vi "Move Window (hwnd).vi"(8 "error in (no error)":errorcluster, 9 "New Position (0,0)":cluster{"left":i16, "top":i16}, 10 "Window Name (\"\")":string, 11 "HWnd":u32) -> (0 "error out":errorcluster, 1 "Prev Position":cluster{"left":i16, "top":i16}, 3 "HWnd Out":u32)   [LabVIEW 2011]
doc: "This function will move the window named in the 'window name' input or identified by the 'window refnum' from its present location to that defined in the 'new position' cluster. Coordinates are pixels relative to upper left corner of the screen.\n\nIf the function is successful, then:\n'window refnum out' = 'window refnum' if window refnum in is valid;\n'window refnum out' is a new window refnum if 'window refnum' is not valid and 'window name' a valid name for a window.\n\nIf the window cannot be found, an error will be returned and window refnum out will be 'Not a Valid Window RefNum'."
uses:
  user32.dll
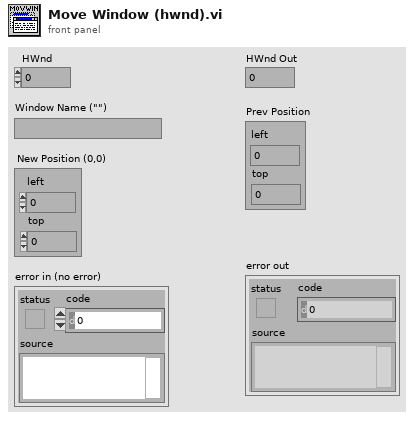
[diagram p1: front panel]
types:
  T1 = typedef "Window Rectangle (hwnd).ctl" = cluster{"left":i16, "top":i16, "right":i16, "bottom":i16}
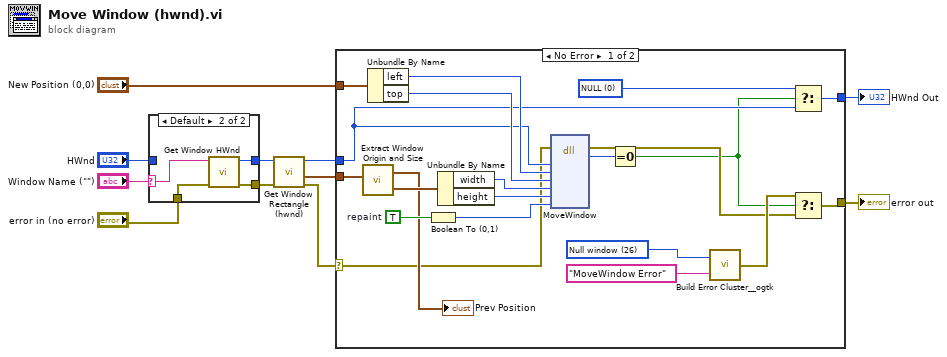
[diagram p0: block diagram]
diagram:
  n1 = case shown="Default" "Window Name (\"\")" {
    selector: "Window Name (\"\")" -> [_ w14]
    tunnel: "error in (no error)" -> [w12 w16]
    tunnel: [w13 w17] -> w3
    tunnel: "HWnd" -> [w13 _]
    tunnel: [w12 w15] -> w7
    frame "" {
    }
    frame Default {
      n2 = call "Get Window HWnd.vi"("error in (no error)"=w16, "Window Name"=w14) -> ("error out"=w15:errorcluster, "HWnd Out"=w17:u32)  [unwired: 8 in]
    }
  }
  n3 = call "Get Window Rectangle (hwnd).vi"("error in (no error)"=w7, "HWnd"=w3) -> ("error out"=w2:errorcluster, "Window Rect"=w11:T1, "HWnd Out"=w4:u32)  [unwired: 7 in]
  n4 = case shown="No Error" w2 {
    selector: w2 -> [w24 w39]
    tunnel: w11 -> [w29 _]
    tunnel: [w20 w39] -> w6
    tunnel: w4 -> [w26 w40]
    tunnel: [w28 w40] -> w5
    tunnel: "New Position (0,0)" -> [w25 _]
    frame No Error {
      w23 = 26 items=["No error", "Argument error", "Memory is full", "Out of zone", "End of file", "File already open", "Generic file I/O error", "File not found", "File permission error", "Disk is full", "Duplicate path", "Too many files open", "System feature not enabled", "Resource file not found", "Cannot add resource", "Resource not found", "Image not found", "Image memory error", "Pen does not exist", "Config type invalid", "Config token not found", "Config parse error", "Config memory error", "Bad external code format", "Bad external code offset", "External code not present", "Null window", "Destroy window error", "Null menu", "Print aborted", "Bad print record", "Print driver error", "Windows error during printing", "Memory error during printing", "Print dialog error", "Generic print error", "Invalid device refnum", "Device not found", "Device parameter error", "Device unit error", "Cannot open device", "Device call aborted", "Generic error", "Cancelled by user", "Object ID too low", "Object ID too high", "Object not in heap", "Unknown heap", "Unknown object (invalid DefProc)", "Unknown object (DefProc not in table)", "Message out of range", "Invalid (null) method", "Unknown message", "Manager call not supported", "Bad address", "Network operation in progress", "Network operation timed out", "Connection is busy", "Network attribute not supported", "Network error", "Address in use", "System out of memory", "Connection aborted", "Connection refused", "Not connected", "Already connected", "Connection closed", "Initialization error (interapplication manager)", "Bad occurrence", "Wait on unbound occurrence handler", "Occurrence queue overflow", "Datalog type conflict", "Unused", "Unrecognized type (interapplication manager)", "Memory corrupt", "Failed to make temporary DLL", "Old CIN version", "Drag socket not found", "Failed to load drop-object", "Failed to register OLE object", "Failed to release OLE object", "Format specifier type mismatch", "Unknown format specifier", "Too few format specifiers", "Too many format specifiers", "Scan failed", "Newer CIN version", "Error converting to variant", "Runtime menu error", "Password tampered", "Variant attribute not found", "Incompatible variant data type", "Event data is not available", "Event Store is not present", "Occurrence is not found", "Event Queue is not created", "Event info is not available", "Refnum passed is NULL", "Error retrieving Class GUID", "Error retrieving CoClass GUID", "Error retrieving TypeLib GUID.", "Bad built application magic bytes.", "Specific driver is different from the specific driver associated with the Logical Name.", "There is no session opened to the class driver.", "Max Error", "MAX - Error with config objects", "MAX - Error loading configuration", "MAX - Group not supported"]
      w27 = u32 0 items=["NULL"]
      w35 = TRUE  # repaint
      n5 = call "Extract Window Origin and Size.vi"("window rect"=w29) -> ("window origin"=→"Prev Position":cluster{"left":i16, "top":i16}, "window size"=w36:cluster{"width":i16, "height":i16})
      n6 = Unbundle By Name(w25) -> ("left"=w38:i16, "top"=w37:i16)
      n7 = Boolean To (0,1)(Boolean=w35) -> (0, 1=w34:i16)
      n8 = Unbundle By Name(w36) -> ("width"=w33:i16, "height"=w32:i16)
      n9 = dll-call lib="USER32.DLL" fn="MoveWindow"(error in=w24, "hWnd"=w26, "left"=w38, "top"=w37, "right"=w33, "bottom"=w32, "repaint"=w34) -> (error out=w19:errorcluster, "error"=w31:i32)  [unwired: 3 in, 6 out]
      n10 = Equal To 0?(x=w31) -> (x = 0?=w18:bool)
      n11 = call <userlib>:"Build Error Cluster__ogtk.vi"("String to Prepend to source (\"\")"="MoveWindow Error" ("String to Prepend to source (\"\")"), "code"=w23) -> ("error out"=w21:errorcluster)
      n12 = Select(t=w27, s=w18, f=w26) -> (s? t:f=w28:u32)
      n13 = Select(t=w21, s=w18, f=w19) -> (s? t:f=w20:errorcluster)
    }
    frame Error {
    }
  }
  "error out" <- w6
  "HWnd Out" <- w5
